vi "Write_Class_Power_Supply.vi"(8 "error in (no error)":errorcluster caption="entrée d'erreur (pas d'erreur)", 10 "Power_Supply (Default)":refnum<class "Power_Supply (Default).lvclass">, 11 "Class Instrument Multimeter en entrée":refnum<class "Class Instrument Power_Supply.lvclass">) -> (0 "error out":errorcluster caption="sortie d'erreur", 3 "Class Instrument Multimeter en sortie":refnum<class "Class Instrument Power_Supply.lvclass">)   [LabVIEW 2020, in "Library Instrument & Equipement.lvlib" / "Library Instruments.lvlib" / "Class Instrument Power_Supply.lvclass"]
uses:
  Class Instrument Power_Supply.lvclass
  Power_Supply/Power_Supply (Default)/Power_Supply (Default).lvclass
  Class Instrument Power_Supply.lvclass/Class Instrument Power_Supply.ctl
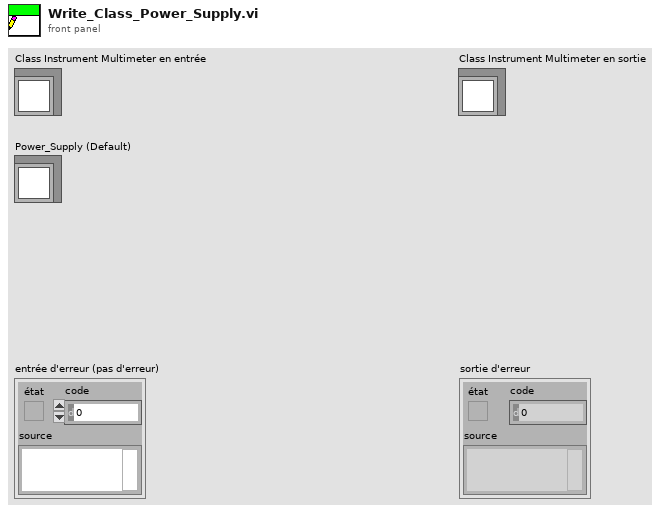
[diagram p1: front panel]
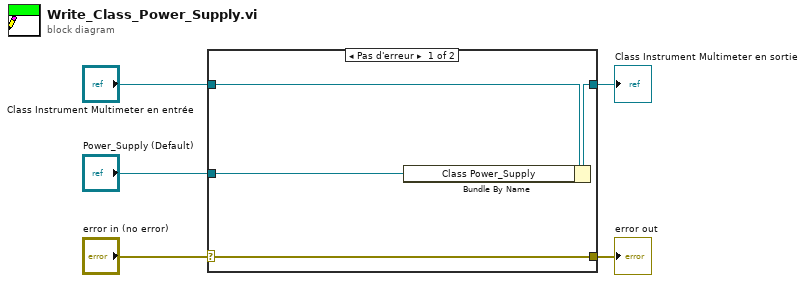
[diagram p0: block diagram]
diagram:
  n1 = case shown="Pas d'erreur" "error in (no error)" {
    selector: "error in (no error)" -> [w9 w10]
    tunnel: [w9 w10] -> w4
    tunnel: [w7 w11] -> w2
    tunnel: "Class Instrument Multimeter en entrée" -> [w8 w11]
    tunnel: "Power_Supply (Default)" -> [w6 _]
    frame No Error {
      n2 = Bundle By Name(cluster=w8, "Class Power_Supply"=w6) -> (w7:refnum<class "Class Instrument Power_Supply.lvclass">)
    }
    frame Error {
    }
  }
  "error out" <- w4
  "Class Instrument Multimeter en sortie" <- w2
